vi "stack_get_top.vi"(8 "error in (no error)":errorcluster, 11 "Lua in":refnum<class "Lua.lvclass">) -> (0 "error out":errorcluster, 2 "size":i32, 3 "Lua out":refnum<class "Lua.lvclass">)   [LabVIEW 2020, in "Lua for LabVIEW.lvlib" / "Lua.lvclass"]
doc: "Push the value at the specified stack index to the Lua stack."
uses:
  Lua.lvclass
  Lua.lvclass/Lua.ctl
  lib/lua.dll/lua.dll.lvlib
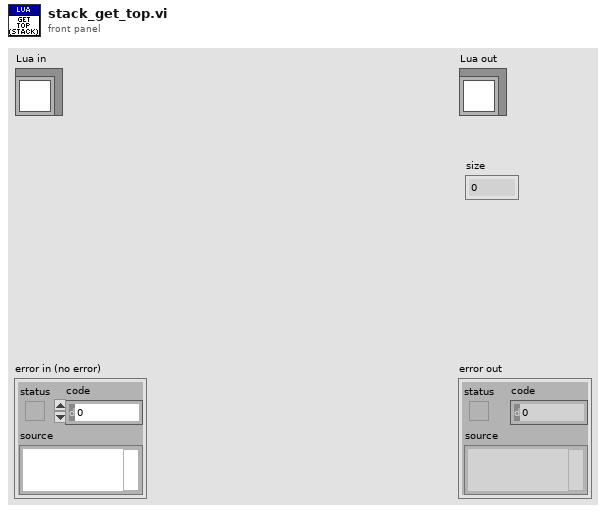
[diagram p1: front panel]
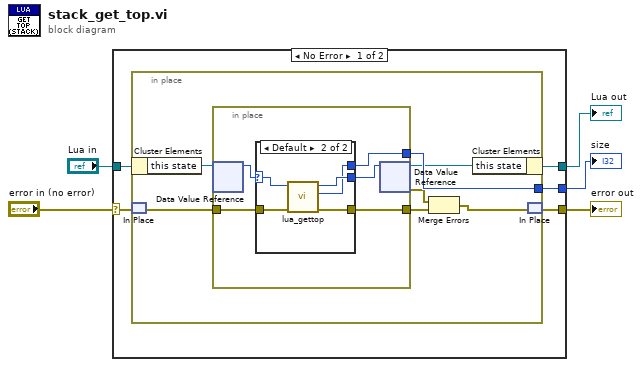
[diagram p0: block diagram]
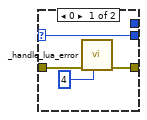
[diagram p2: hidden frame]
diagram:
  n1 = case shown="No Error" "error in (no error)" {
    selector: "error in (no error)" -> [w7 w33]
    tunnel: [w8 w33] -> w4
    tunnel: [w9 w32] -> w2
    tunnel: "Lua in" -> [w10 w32]
    tunnel: [w6 _] -> w1
    frame No Error {
      n2 = in-place {
        in-place-border: [w16] -> w6
        n3 = in-place-cluster #1(w10) -> ("this state"=w15:refnum<data-value>)
        n4 = in-place-match #2(w7) -> (w17:errorcluster)
        n5 = in-place {
          in-place-border: w17 -> [w22]
          in-place-border: [w21] -> w16
          in-place-border: [w18] -> w13
          n6 = in-place-dvr #3(w15) -> (w20:u64)  [unwired: 1 out]
          n7 = case shown="Default" w20 {
            selector: w20 -> [w26 w31]
            tunnel: [w26 w30] -> w19
            tunnel: w22 -> [w23 w28]
            tunnel: [w24 w29] -> w18
            tunnel: [_ w27] -> w21
            frame 0 {
              n8 = call "_handle_lua_error.vi"("lua status"=4 ("lua_load errcode"), "error in (no error)"=w23) -> ("error out"=w24:errorcluster)  [unwired: 9 in]
            }
            frame Default {
              n9 = call "lua_gettop.vi"("error in (no error)"=w28, "lua_state_p"=w31) -> ("error out"=w29:errorcluster, "index"=w27:i32, "lua_state_p out"=w30:u64)  [unwired: 7 in]
            }
          }
          n10 = in-place-dvr #3(w19) -> (w11:refnum<data-value>, w14:errorcluster)
        }
        n11 = Merge Errors(w14, w13) -> (w12:errorcluster)
        n12 = in-place-cluster #1("this state"=w11) -> (w9:refnum<class "Lua.lvclass">)
        n13 = in-place-match #2(w12) -> (w8:errorcluster)
      }
    }
    frame Error {
    }
  }
  "error out" <- w4
  "Lua out" <- w2
  "size" <- w1
